vi "Write Std Out with Redirection.vi"(8 "error in (no error)":errorcluster, 11 "string":string) -> (0 "error out":errorcluster)   [LabVIEW 2015]
uses:
  kernel32.dll
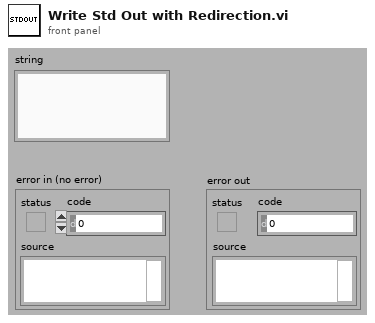
[diagram p1: front panel]
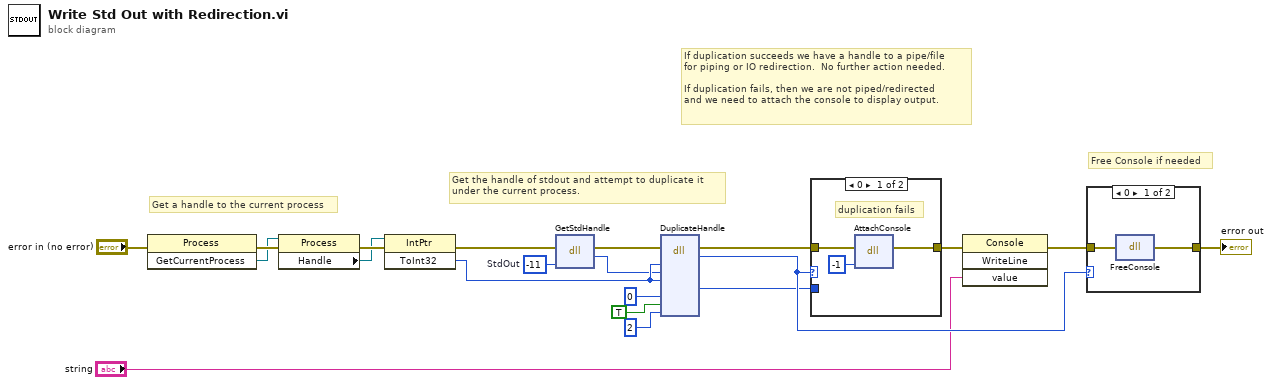
[diagram p0: block diagram]
diagram:
  w11 = -11  # StdOut
  # "If duplication succeeds we have a handle to a pipe/file\nfor piping or IO redirection.  No further action needed.\n\nIf duplication fails, then we are not piped/redirected\nand we need to attach the console to display output."
  # "Free Console if needed"
  # "Get the handle of stdout and attempt to duplicate it\nunder the current process."
  # "Get a handle to the current process"
  n1 = invoke class="Process" method="GetCurrentProcess"(error in="error in (no error)") -> (error out=w18:errorcluster, "GetCurrentProcess"=w9:refnum<k24>)  [unwired: 2 in, 1 out]
  n2 = property class="Process"(reference=w9, error in=w18) -> (error out=w17:errorcluster, "Handle"=w8:refnum<k24>)  [unwired: 1 out]
  n3 = invoke class="IntPtr" method="ToInt32"(reference=w8, error in=w17) -> (error out=w12:errorcluster, "ToInt32"=w19:i32)  [unwired: 1 in, 1 out]
  n4 = dll-call lib="kernel32.dll" fn="GetStdHandle"(error in=w12, "nStdHandle"=w11) -> (error out=w7:errorcluster, "return type"=w10:i32)  [unwired: 3 in, 1 out]
  n5 = dll-call lib="kernel32.dll" fn="DuplicateHandle"(error in=w7, "hSourceProcess"=w19, "hSourceHandle"=w10, "hTargetProcess"=w19, "dwDesirecAccess"=u16 0, "bInheritHandle"=TRUE, "dwOptions"=u16 2) -> (error out=w16:errorcluster, "return type"=w5:u8, "lpTargetHandle"=w4:i32)  [unwired: 9 in, 1 out]
  n6 = case shown="0" w5 {
    tunnel: w16 -> [w23 w24]
    tunnel: [w22 w24] -> w6
    tunnel: w4 -> [_ _]
    frame 0 {
      # "duplication fails"
      n7 = dll-call lib="kernel32.dll" fn="AttachConsole"(error in=w23, "arg1"=-1) -> (error out=w22:errorcluster)  [unwired: 4 in, 1 out]
    }
    frame Default {
      # "duplication succeeds"
    }
  }
  n8 = invoke class="Console" method="WriteLine"(error in=w6, "value"="string") -> (error out=w20:errorcluster)  [unwired: 2 in, 3 out]
  n9 = case shown="0" w5 {
    tunnel: w20 -> [w26 w27]
    tunnel: [w25 w27] -> w3
    frame 0 {
      n10 = dll-call lib="kernel32.dll" fn="FreeConsole"(error in=w26) -> (error out=w25:errorcluster)  [unwired: 2 in, 2 out]
    }
    frame Default {
    }
  }
  "error out" <- w3
